vi "FABR-Plot AvsF.vi"(0 "Analysis":T1, 1 "I-O":refnum<vi>, 11 "error in (no error)":errorcluster) -> (15 "error out":errorcluster)   [LabVIEW 2020]
uses:
  Typedefs/FABR-Analysis State.ctl
  Threshold Estimation VIs/ABR3-Threshold Estimation Result.ctl
  epl-vi-lib/Utility VIs/Math VIs/LinSpace (x0-dx-npts).vi
panel:
  # "Freq X Level X Time"
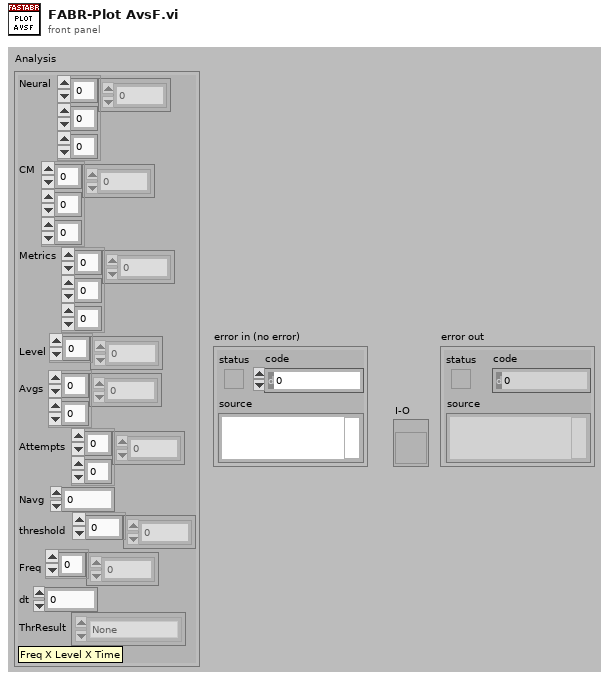
[diagram p1: front panel]
types:
  T1 = typedef "FABR-Analysis State.ctl" = cluster{"Neural":dbl[][][], "CM":dbl[][][], "Metrics":dbl[][][], "Level":dbl[], "Avgs":i32[][], "Attempts":i32[][], "Navg":i32, "threshold":dbl[], "Freq":dbl[], "dt":dbl, "ThrResult":T2[]}
  T2 = typedef "ABR3-Threshold Estimation Result.ctl" = enum16{"None", "Power", "Sigmoid", "Power (noisy)", "Suprathreshold", "Invalid"}
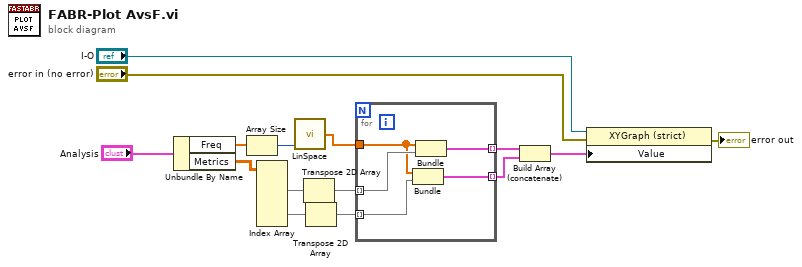
[diagram p0: block diagram]
diagram:
  n1 = Unbundle By Name("Analysis") -> ("Freq"=w3:dbl[], "Metrics"=w11:dbl[][][])
  n2 = Array Size(array=w3) -> (size(s)=w2:i32)
  n3 = Index Array(array=w11) -> (element #1=w10:dbl[][], element #2=w9:dbl[][])  [unwired: 6 in]
  n4 = call-poly "LinSpace.vi"("npts"=w2) -> ("Array"=w1:dbl[])  [unwired: 3 in, 1 out]
  n5 = Transpose 2D Array(2D array=w10) -> (transposed array=w5:dbl[][])
  n6 = Transpose 2D Array(2D array=w9) -> (transposed array=w4:dbl[][])
  n7 = for {
    tunnel: w1 -> [w17]
    tunnel: w5 -> [w19] mode=indexing
    tunnel: [w20] -> w8 mode=indexing
    tunnel: w4 -> [w18] mode=indexing
    tunnel: [w16] -> w7 mode=indexing
    n8 = Bundle("Array"=w17, w18) -> (w16:cluster{"Array":dbl[], dbl[]})  [unwired: 1 in]
    n9 = Bundle("Array"=w17, w19) -> (w20:cluster{"Array":dbl[], dbl[]})  [unwired: 1 in]
  }
  n10 = Build Array (concatenate)(w8, w7) -> (w6:cluster{"Array":dbl[], dbl[]}[])
  n11 = property class="XYGraph (strict)"(reference="I-O", error in="error in (no error)", "Value"=w6) -> (error out=→"error out":errorcluster)  [unwired: 1 out]
